vi "CRYDelay waveform for best match.vi"(4 "Sampling rate (Hz)":i32=1000, 10 "stimulus waveform":dbl[](array[numeric]), 11 "Recorded waveform":dbl[](array[numeric]) format="%.2f") -> (0 "Polarity Value":dbl, 1 "Delay Samples":i32, 2 "Delay (ms)":dbl format="%.2f", 3 "Delayed waveform":dbl[](array[numeric]) format="%.2f", 5 "Polarity Amplitude":dbl, 7 "Polarity Time":dbl)   [LabVIEW 2013]
panel:
  out "T0":dbl
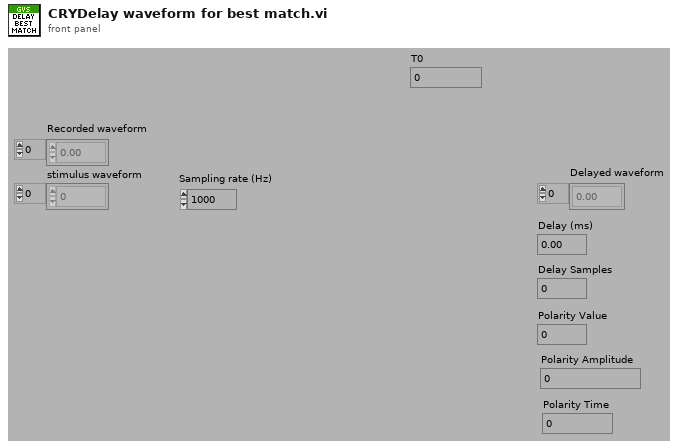
[diagram p1: front panel]
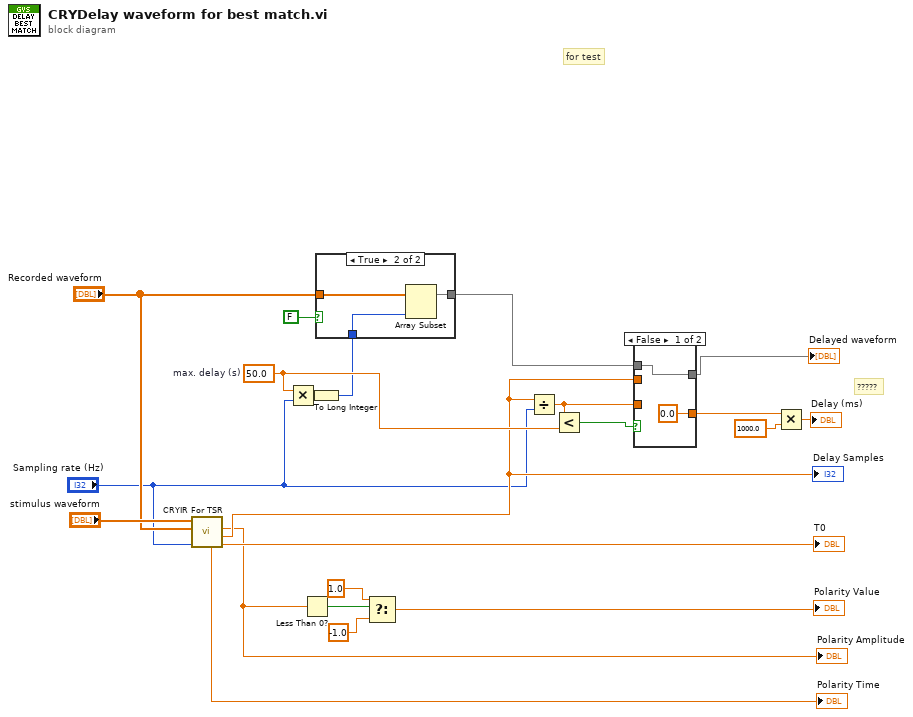
[diagram p0: block diagram]
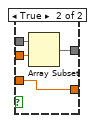
[diagram p3: hidden frame]
diagram:
  w20 = 50.0  # max. delay (s)
  # "?????"
  # "for test"
  n1 = call "CRYIR For TSR.vi"("Fs"="Sampling rate (Hz)", "Response[y(t)]"="Recorded waveform", "Stimulus[x(t)]"="stimulus waveform") -> ("T0"=→"T0":dbl, "T max Index"=w9:dbl, "T max Amplitude"=w6:dbl, "T max Time"=→"Polarity Time":dbl)  [unwired: 4 in, 1 out]
  "Delay Samples" <- w9
  "Polarity Amplitude" <- w6
  n2 = Multiply(x=w20, y="Sampling rate (Hz)") -> (x*y=w21:dbl)
  n3 = Less Than 0?(x=w6) -> (x < 0?=w5:bool)
  n4 = To Long Integer(number=w21) -> (32bit integer=w16:i32)
  n5 = case shown="True" FALSE {
    tunnel: w16 -> [_ w24]
    tunnel: "Recorded waveform" -> [w23 w26]
    tunnel: [w23 w25] -> w13
    frame False {
    }
    frame True {
      n6 = Array Subset(array=w26, length=w24) -> (w25:dbl[])  [unwired: 1 in]
    }
  }
  n7 = Select(t=1.0, s=w5, f=-1.0 ("t")) -> (s? t:f=→"Polarity Value":dbl)
  n8 = Divide(x=w9, y="Sampling rate (Hz)") -> (x/y=w22:dbl)
  n9 = Less?(x=w22, y=w20) -> (x < y?=w8:bool)
  n10 = case shown="False" w8 {
    tunnel: w9 -> [_ w32]
    tunnel: w13 -> [w28 w31]
    tunnel: [w28 w30] -> w18
    tunnel: w22 -> [_ w29]
    tunnel: [0.0 w29] -> w17
    frame False {
    }
    frame True {
      n11 = Array Subset(array=w31, index=w32) -> (w30:dbl[])  [unwired: 1 in]
    }
  }
  "Delayed waveform" <- w18
  n12 = Multiply(x=w17, y=1000.0) -> (x*y=→"Delay (ms)":dbl)
